vi "Register PVs.vi"(8 "error in (no error)":errorcluster, 10 "Activate?":bool, 11 "CS++ControllerActor in":refnum<class "CS++ControllerActor.lvclass">) -> (0 "error out":errorcluster, 3 "CS++ControllerActor out":refnum<class "CS++ControllerActor.lvclass">)   [LabVIEW 2014, in "CS++ControllerActor.lvlib" / "CS++ControllerActor.lvclass"]
uses:
  CS++ControllerActor.lvclass
  CS++ControllerActor.lvclass/CS++ControllerActor.ctl
  CS++PVMonitor Messages/Register PVs Msg/Register PVs Msg.lvclass/Register PVs Msg.ctl
  <vilib>/ActorFramework/Message Enqueuer/Message Enqueuer.lvclass/Message Enqueuer.ctl
  <vilib>/ActorFramework/Message Enqueuer/Enqueue.vi
  <vilib>/ActorFramework/Message Priority Queue/Priority Enqueue.vi
  <vilib>/ActorFramework/Message Enqueuer/Message Enqueuer.lvclass
  CS++PVMonitor Messages/CS++PVUpdate Msg/CS++PVUpdate Msg.lvclass
  CS++PVMonitor Messages/Register PVs Msg/Register PVs Msg.lvclass
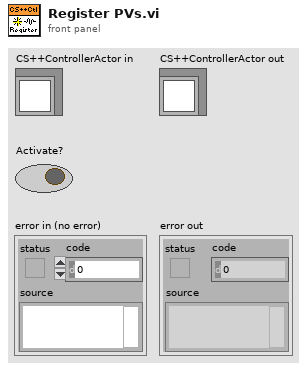
[diagram p1: front panel]
types:
  T1 = cluster{"Accessors:Device Actor's Enqueuer":refnum<class "Message Enqueuer.lvclass">, "Msgs":refnum<class "CS++PVUpdate Msg.lvclass">[]}[]
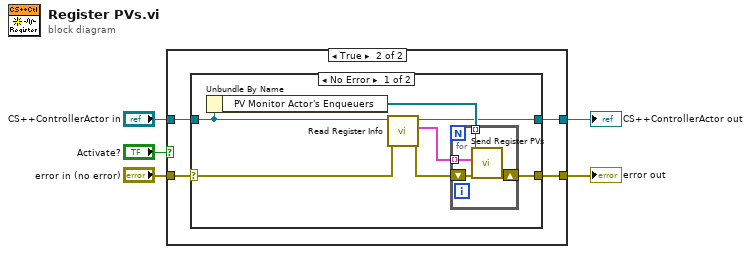
[diagram p0: block diagram]
diagram:
  n1 = case shown="True" "Activate?" {
    tunnel: "error in (no error)" -> [w6 w11]
    tunnel: [w6 w10] -> w4
    tunnel: "CS++ControllerActor in" -> [w7 w9]
    tunnel: [w7 w8] -> w2
    frame False {
    }
    frame True {
      n2 = case shown="No Error" w11 {
        selector: w11 -> [w13 w24]
        tunnel: [w12 w24] -> w10
        tunnel: [w16 w23] -> w8
        tunnel: w9 -> [w17 w23]
        frame No Error {
          n3 = Unbundle By Name(w17) -> ("PV Monitor Actor's Enqueuers"=w18:refnum<class "Message Enqueuer.lvclass">[])
          n4 = call "Read Register Info.vi"("error in (no error)"=w13, "CS++ControllerActor in"=w17) -> ("error out"=w14:errorcluster, "Register Info"=w15:T1, "CS++ControllerActor out"=w16:refnum<class "CS++ControllerActor.lvclass">)  [unwired: 7 in]
          n5 = for {
            tunnel: w18 -> [w22] mode=indexing
            tunnel: w15 -> [w21] mode=indexing
            shift-right: [w19] -> w12
            shift-left: w14 -> [w20]
            n6 = call "Send Register PVs.vi"("error in (no error)"=w20, "Register Info"=w21, "Message Enqueuer"=w22) -> ("error out"=w19:errorcluster)  [unwired: 7 in, 1 out]
          }
        }
        frame Error {
        }
      }
    }
  }
  "error out" <- w4
  "CS++ControllerActor out" <- w2
